vi "WriteConfiguration.vi"(8 "error in":errorcluster) -> (0 "error out":errorcluster)   [LabVIEW 2012]
uses:
  GlobalVariables/SystemParameters.vi
  GlobalVariables/LanguagesSettings.vi
  GlobalVariables/StabilizationSettings.vi
  GlobalVariables/PT02Parameters.vi
  GlobalVariables/PT01Parameters.vi
  <vilib>/Utility/config.llb/Write Key (U32).vi
  <vilib>/Utility/config.llb/Write Key (String).vi
  <vilib>/Utility/config.llb/Write Key (I32).vi
  <vilib>/Utility/config.llb/Write Key (Double).vi
  <vilib>/Utility/config.llb/NI_LVConfig.lvlib
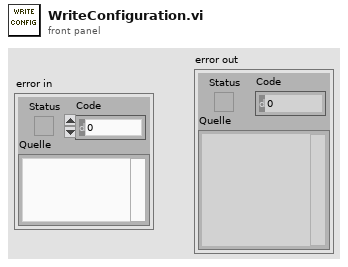
[diagram p1: front panel]
types:
  T1 = cluster{"baudrate":u32, "databits":u16, "paritybit":u16, "stopbits":u16, "flux control":u16, "Port":string, "Register Address":u16, "Serial Parameters":cluster{"Mode":enum16{"RTU", "ASCII"}, "Slave Address":u8}, "Timeout":u32, "PressureLimit":dbl}
  T2 = typedef "NI_LVConfig.lvlib/Config Data RefNum.ctl" = refnum<k1>
  T3 = cluster{"defaultLanguage":string, "languageFile":string, "languages":string, "HardwarePresent":bool}
  T4 = cluster{"SupportedLanguagesList":string[], "ActiveLanguage":string, "ActiveLanguageIndex":u16, "LocalisationFileContent[out]":cluster{"Indices":u32[], "LocalizedWords":string[][]}}
  T5 = cluster{"MinimalWaitTime":u32, "VarianceTrigger":dbl, "MaxWaitTime":u32}
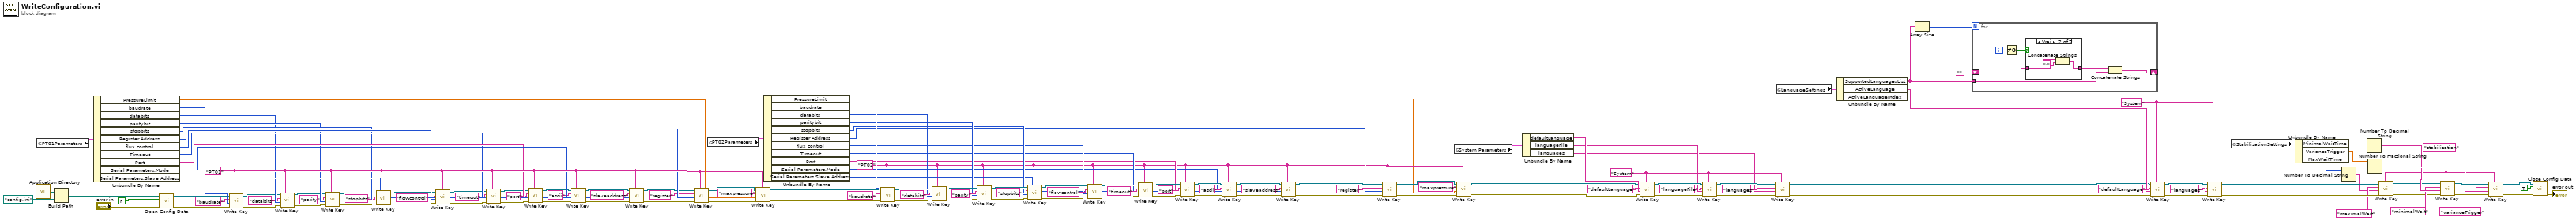
[diagram p0: block diagram]
diagram:
  w47 = "PT01" ("section")
  w54 = "stabilization" ("section")
  w81 = "System"
  w94 = "System"
  w60 = "PT02" ("section")
  n1 = call <vilib>:"Application Directory.vi"() -> ("Application Directory"=w142:path)
  n2 = global read "PT01Parameters.vi" "PT01Parameters"() -> (w5:T1)
  n3 = Build Path(base path=w142, name or relative path=path "config.ini" ("configuration file path")) -> (appended path=w140:path)
  n4 = Unbundle By Name(w5) -> ("PressureLimit"=w48:dbl, "baudrate"=w34:u32, "databits"=w35:u16, "paritybit"=w36:u16, "stopbits"=w37:u16, "Register Address"=w43:u16, "flux control"=w38:u16, "Timeout"=w39:u32, "Port"=w40:string, "Serial Parameters.Mode"=w41:enum16{"RTU", "ASCII"}, "Serial Parameters.Slave Address"=w42:u8)
  n5 = call <vilib>:"Open Config Data.vi"("error in (no error)"="error in", "create file if necessary (T)"=FALSE ("create file if necessary? (T)"), "configuration file path"=w140) -> ("error out"=w1:errorcluster, "refnum"=w2:T2)  [unwired: 6 in, 1 out]
  n6 = call-poly <vilib>:"Write Key.vi"("section"=w47, "error in (no error)"=w1, "value"=w34, "key"="baudrate", "refnum"=w2) -> ("error out"=w7:errorcluster, "refnum out"=w10:T2)  [unwired: 4 in, 1 out]
  n7 = call-poly <vilib>:"Write Key.vi"("section"=w47, "error in (no error)"=w7, "value"=w35, "key"="databits", "refnum"=w10) -> ("error out"=w6:errorcluster, "refnum out"=w11:T2)  [unwired: 4 in, 1 out]
  n8 = call-poly <vilib>:"Write Key.vi"("section"=w47, "error in (no error)"=w6, "value"=w36, "key"="parity", "refnum"=w11) -> ("error out"=w17:errorcluster, "refnum out"=w12:T2)  [unwired: 4 in, 1 out]
  n9 = call-poly <vilib>:"Write Key.vi"("section"=w47, "error in (no error)"=w17, "value"=w37, "key"="stopbits", "refnum"=w12) -> ("error out"=w18:errorcluster, "refnum out"=w13:T2)  [unwired: 4 in, 1 out]
  n10 = call-poly <vilib>:"Write Key.vi"("section"=w47, "error in (no error)"=w18, "value"=w38, "key"="flowcontrol", "refnum"=w13) -> ("error out"=w19:errorcluster, "refnum out"=w14:T2)  [unwired: 4 in, 1 out]
  n11 = call-poly <vilib>:"Write Key.vi"("section"=w47, "error in (no error)"=w19, "value"=w39, "key"="timeout", "refnum"=w14) -> ("error out"=w20:errorcluster, "refnum out"=w15:T2)  [unwired: 4 in, 1 out]
  n12 = call-poly <vilib>:"Write Key.vi"("section"=w47, "error in (no error)"=w20, "value"=w40, "key"="port", "refnum"=w15) -> ("error out"=w21:errorcluster, "refnum out"=w16:T2)  [unwired: 4 in, 1 out]
  n13 = call-poly <vilib>:"Write Key.vi"("section"=w47, "error in (no error)"=w21, "value"=w41, "key"="ascii", "refnum"=w16) -> ("error out"=w22:errorcluster, "refnum out"=w23:T2)  [unwired: 4 in, 1 out]
  n14 = call-poly <vilib>:"Write Key.vi"("section"=w47, "error in (no error)"=w22, "value"=w42, "key"="slaveaddress", "refnum"=w23) -> ("error out"=w30:errorcluster, "refnum out"=w31:T2)  [unwired: 4 in, 1 out]
  n15 = call-poly <vilib>:"Write Key.vi"("section"=w47, "error in (no error)"=w30, "value"=w43, "key"="register", "refnum"=w31) -> ("error out"=w45:errorcluster, "refnum out"=w46:T2)  [unwired: 4 in, 1 out]
  n16 = global read "PT02Parameters.vi" "PT02Parameters"() -> (w139:T1)
  n17 = call-poly <vilib>:"Write Key.vi"("section"=w47, "error in (no error)"=w45, "value"=w48, "key"="maxpressure", "refnum"=w46) -> ("error out"=w4:errorcluster, "refnum out"=w3:T2)  [unwired: 4 in, 1 out]
  n18 = Unbundle By Name(w139) -> ("PressureLimit"=w59:dbl, "baudrate"=w110:u32, "databits"=w109:u16, "paritybit"=w108:u16, "stopbits"=w107:u16, "Register Address"=w101:u16, "flux control"=w106:u16, "Timeout"=w105:u32, "Port"=w104:string, "Serial Parameters.Mode"=w103:enum16{"RTU", "ASCII"}, "Serial Parameters.Slave Address"=w102:u8)
  n19 = call-poly <vilib>:"Write Key.vi"("section"=w60, "error in (no error)"=w4, "value"=w110, "key"="baudrate", "refnum"=w3) -> ("error out"=w137:errorcluster, "refnum out"=w134:T2)  [unwired: 4 in, 1 out]
  n20 = call-poly <vilib>:"Write Key.vi"("section"=w60, "error in (no error)"=w137, "value"=w109, "key"="databits", "refnum"=w134) -> ("error out"=w138:errorcluster, "refnum out"=w133:T2)  [unwired: 4 in, 1 out]
  n21 = call-poly <vilib>:"Write Key.vi"("section"=w60, "error in (no error)"=w138, "value"=w108, "key"="parity", "refnum"=w133) -> ("error out"=w127:errorcluster, "refnum out"=w132:T2)  [unwired: 4 in, 1 out]
  n22 = call-poly <vilib>:"Write Key.vi"("section"=w60, "error in (no error)"=w127, "value"=w107, "key"="stopbits", "refnum"=w132) -> ("error out"=w126:errorcluster, "refnum out"=w131:T2)  [unwired: 4 in, 1 out]
  n23 = call-poly <vilib>:"Write Key.vi"("section"=w60, "error in (no error)"=w126, "value"=w106, "key"="flowcontrol", "refnum"=w131) -> ("error out"=w125:errorcluster, "refnum out"=w130:T2)  [unwired: 4 in, 1 out]
  n24 = call-poly <vilib>:"Write Key.vi"("section"=w60, "error in (no error)"=w125, "value"=w105, "key"="timeout", "refnum"=w130) -> ("error out"=w124:errorcluster, "refnum out"=w129:T2)  [unwired: 4 in, 1 out]
  n25 = call-poly <vilib>:"Write Key.vi"("section"=w60, "error in (no error)"=w124, "value"=w104, "key"="port", "refnum"=w129) -> ("error out"=w123:errorcluster, "refnum out"=w128:T2)  [unwired: 4 in, 1 out]
  n26 = call-poly <vilib>:"Write Key.vi"("section"=w60, "error in (no error)"=w123, "value"=w103, "key"="ascii", "refnum"=w128) -> ("error out"=w122:errorcluster, "refnum out"=w121:T2)  [unwired: 4 in, 1 out]
  n27 = call-poly <vilib>:"Write Key.vi"("section"=w60, "error in (no error)"=w122, "value"=w102, "key"="slaveaddress", "refnum"=w121) -> ("error out"=w114:errorcluster, "refnum out"=w113:T2)  [unwired: 4 in, 1 out]
  n28 = call-poly <vilib>:"Write Key.vi"("section"=w60, "error in (no error)"=w114, "value"=w101, "key"="register", "refnum"=w113) -> ("error out"=w64:errorcluster, "refnum out"=w61:T2)  [unwired: 4 in, 1 out]
  n29 = global read "SystemParameters.vi" "System Parameters"() -> (w99:T3)
  n30 = call-poly <vilib>:"Write Key.vi"("section"=w60, "error in (no error)"=w64, "value"=w59, "key"="maxpressure", "refnum"=w61) -> ("error out"=w63:errorcluster, "refnum out"=w62:T2)  [unwired: 4 in, 1 out]
  n31 = Unbundle By Name(w99) -> ("defaultLanguage"=w92:string, "languageFile"=w91:string, "languages"=w88:string)
  n32 = call-poly <vilib>:"Write Key.vi"("section"=w94, "error in (no error)"=w63, "value"=w92, "key"="defaultLanguage", "refnum"=w62) -> ("error out"=w96:errorcluster, "refnum out"=w97:T2)  [unwired: 4 in, 1 out]
  n33 = call-poly <vilib>:"Write Key.vi"("section"=w94, "error in (no error)"=w96, "value"=w91, "key"="languageFile", "refnum"=w97) -> ("error out"=w95:errorcluster, "refnum out"=w98:T2)  [unwired: 4 in, 1 out]
  n34 = call-poly <vilib>:"Write Key.vi"("section"=w94, "error in (no error)"=w95, "value"=w88, "key"="languages", "refnum"=w98) -> ("error out"=w49:errorcluster, "refnum out"=w50:T2)  [unwired: 4 in, 1 out]
  n35 = global read "LanguagesSettings.vi" "LanguageSettings"() -> (w87:T4)
  n36 = Unbundle By Name(w87) -> ("SupportedLanguagesList"=w84:string[], "ActiveLanguage"=w79:string)  [unwired: 1 out]
  n37 = Array Size(array=w84) -> (size(s)=w86:i32)
  n38 = for {
    N: w86 -> [_]
    shift-right: [w148] -> w78
    shift-left: "" -> [w147]
    tunnel: w84 -> [w151] mode=indexing
    i -> [w149]
    n39 = Not Equal To 0?(x=w149) -> (x != 0?=w150:bool)
    n40 = case shown="Vrai" w150 {
      tunnel: w147 -> [w152 w154]
      tunnel: [w152 w153] -> w146
      frame False {
      }
      frame True {
        n41 = Concatenate Strings(w154, ";") -> (w153:string)
      }
    }
    n42 = Concatenate Strings(w146, w151) -> (w148:string)
  }
  n43 = call-poly <vilib>:"Write Key.vi"("section"=w81, "error in (no error)"=w49, "value"=w79, "key"="defaultLanguage", "refnum"=w50) -> ("error out"=w82:errorcluster, "refnum out"=w83:T2)  [unwired: 4 in, 1 out]
  n44 = call-poly <vilib>:"Write Key.vi"("section"=w81, "error in (no error)"=w82, "value"=w78, "key"="languages", "refnum"=w83) -> ("error out"=w57:errorcluster, "refnum out"=w56:T2)  [unwired: 4 in, 1 out]
  n45 = global read "StabilizationSettings.vi" "StabilizationSettings"() -> (w72:T5)
  n46 = Unbundle By Name(w72) -> ("MinimalWaitTime"=w71:u32, "VarianceTrigger"=w70:dbl, "MaxWaitTime"=w52:u32)
  n47 = Number To Decimal String(number=w52) -> (decimal integer string=w51:string)  [unwired: 1 in]
  n48 = Number To Decimal String(number=w71) -> (decimal integer string=w68:string)  [unwired: 1 in]
  n49 = Number To Fractional String(number=w70) -> (F-format string=w69:string)  [unwired: 3 in]
  n50 = call-poly <vilib>:"Write Key.vi"("section"=w54, "error in (no error)"=w57, "value"=w51, "key"="maximalWait", "refnum"=w56) -> ("error out"=w58:errorcluster, "refnum out"=w55:T2)  [unwired: 4 in, 1 out]
  n51 = call-poly <vilib>:"Write Key.vi"("section"=w54, "error in (no error)"=w58, "value"=w68, "key"="minimalWait", "refnum"=w55) -> ("error out"=w76:errorcluster, "refnum out"=w74:T2)  [unwired: 4 in, 1 out]
  n52 = call-poly <vilib>:"Write Key.vi"("section"=w54, "error in (no error)"=w76, "value"=w69, "key"="varianceTrigger", "refnum"=w74) -> ("error out"=w75:errorcluster, "refnum out"=w73:T2)  [unwired: 4 in, 1 out]
  n53 = call <vilib>:"Close Config Data.vi"("error in (no error)"=w75, "write file if changed (T)"=TRUE ("create file if necessary? (T)"), "refnum"=w73) -> ("error out"=→"error out":errorcluster)  [unwired: 7 in, 1 out]
